vi "ActionVIOnLoad.vi"(8 "error in (no error)":errorcluster, 11 "Device Item Ref in":T1 format="%.0x") -> (0 "error out":errorcluster, 3 "Device Item Ref out":T1 format="%.0x")   [LabVIEW 2019, in "Ghost Bus Addon System Explorer.lvlib"]
uses:
  Ghost Bus Addon System Explorer.lvlib
  NationalInstruments.VeriStand.SystemDefinitionAPI
  Addon Shared/SubVIs/GUID Lookup.vi
  Addon Shared/Ghost Bus Addon Shared.lvlib
  <vilib>/NI/NI VeriStand Advanced SysDef API/SysDef API/Advanced System Definition.lvlib
  <vilib>/NI VeriStand/Custom Device API/Custom Device Item Ref.ctl
  <vilib>/NI VeriStand/Custom Device API/Custom Device API.lvlib
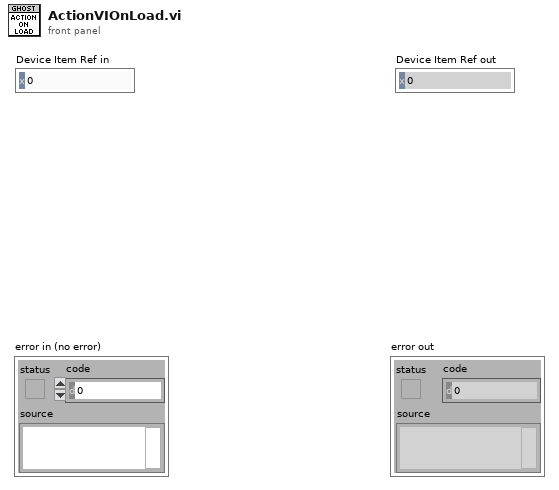
[diagram p1: front panel]
types:
  T1 = typedef "Custom Device API.lvlib/Custom Device Item Ref.ctl" = u64
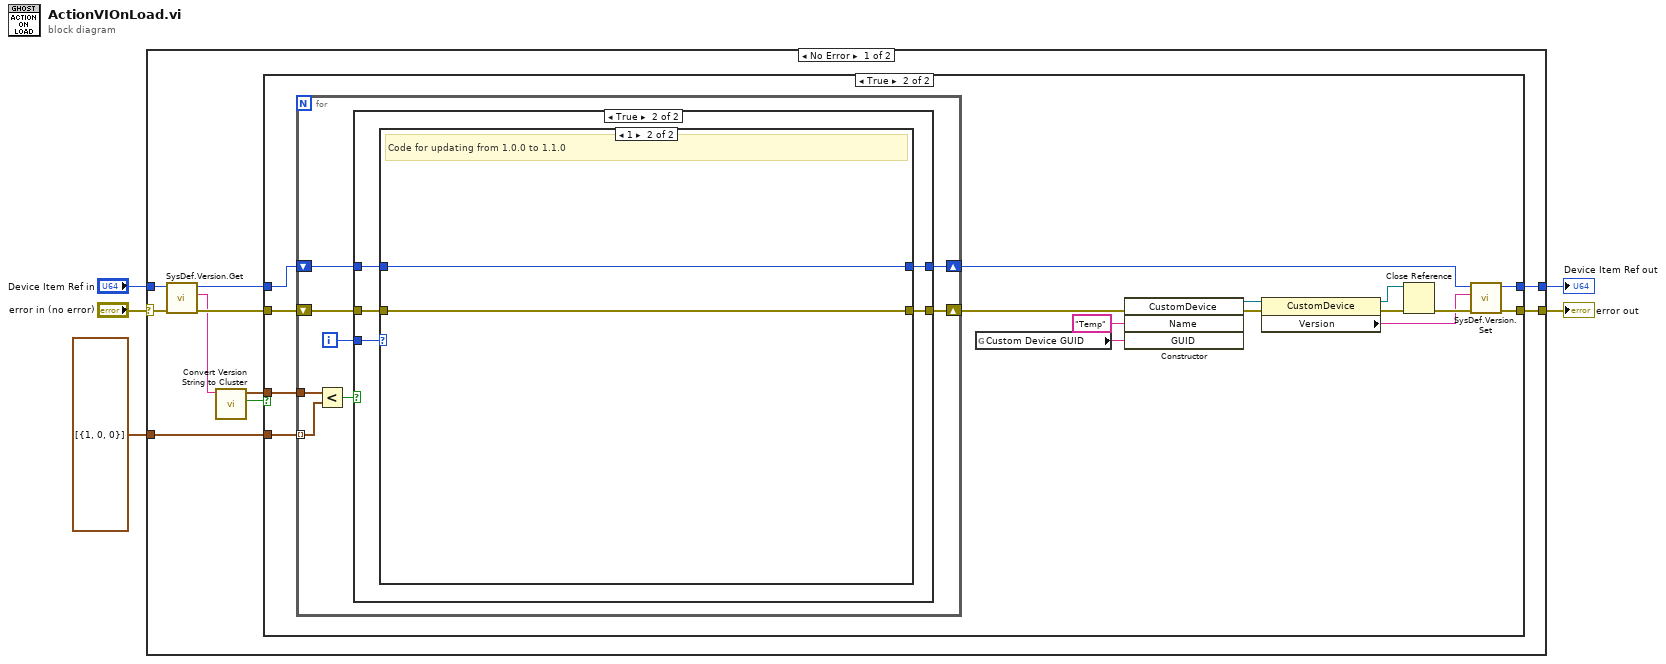
[diagram p0: block diagram]
diagram:
  n1 = case shown="No Error" "error in (no error)" {
    selector: "error in (no error)" -> [w12 w54]
    tunnel: [w14 w54] -> w4
    tunnel: "Device Item Ref in" -> [w11 w53]
    tunnel: [w13 w53] -> w2
    tunnel: cluster{i32, i32, i32}[] [{1, 0, 0}] -> [w15 _]
    frame No Error {
      n2 = call <vilib>:"SysDef.Version.Get.vi"("error in (no error)"=w12, "nodeID"=w11) -> ("error out"=w10:errorcluster, "Version"=w8:string, "nodeID out"=w9:u64)  [unwired: 7 in]
      n3 = call "Convert Version String to Cluster.vi"("Version"=w8) -> ("Version Valid?"=w6:bool, "Version"=w7:cluster{i32, i32, i32})  [unwired: 9 in]
      n4 = case shown="True" w6 {
        tunnel: w15 -> [_ w25]
        tunnel: [w16 w23] -> w14
        tunnel: [w17 w21] -> w13
        tunnel: w10 -> [w16 w20]
        tunnel: w9 -> [w17 w19]
        tunnel: w7 -> [_ w18]
        frame False {
        }
        frame True {
          n5 = for {
            tunnel: w25 -> [w36] mode=indexing
            shift-right: [w40] -> w24
            shift-left: w20 -> [w34]
            shift-right: [w39] -> w26
            shift-left: w19 -> [w35]
            tunnel: w18 -> [w37]
            i -> [w38]
            n6 = Less?(x=w37, y=w36) -> (x < y?=w41:bool)
            n7 = case shown="True" w41 {
              tunnel: w34 -> [w43 w48]
              tunnel: w35 -> [w42 w47]
              tunnel: [w43 w45] -> w40
              tunnel: [w42 w46] -> w39
              tunnel: w38 -> [_ w44]
              frame False {
              }
              frame True {
                n8 = case shown="1" w44 {
                  tunnel: w48 -> [w49 w52]
                  tunnel: w47 -> [w50 w51]
                  tunnel: [w50 w51] -> w46
                  tunnel: [w49 w52] -> w45
                  frame Default {
                  }
                  frame 1 {
                    # "Code for updating from 1.0.0 to 1.1.0"
                  }
                }
              }
            }
          }
          n9 = global read "GUID Lookup.vi" "Custom Device GUID"() -> (w22:string)
          n10 = constructor class="CustomDevice"(error in=w24, "Name"="Temp", "GUID"=w22) -> (reference out=w33:refnum<k24>, error out=w32:errorcluster)  [unwired: 2 in, 3 out]
          n11 = property class="CustomDevice"(reference=w33, error in=w32) -> (reference out=w30:refnum<k24>, error out=w31:errorcluster, "Version"=w28:string)
          n12 = Close Reference(reference=w30, error in (no error)=w31) -> (error out=w29:errorcluster)
          n13 = call <vilib>:"SysDef.Version.Set.vi"("error in (no error)"=w29, "Version"=w28, "nodeID"=w26) -> ("error out"=w23:errorcluster, "nodeID out"=w21:u64)  [unwired: 7 in]
        }
      }
    }
    frame Error {
    }
  }
  "error out" <- w4
  "Device Item Ref out" <- w2
